vi "SVT Send Data to Waterfall for Octave.vi"(0 "waterfall ref":refnum<vi>, 1 "axis labels":T1, 5 "octave spectra":T6(array[cluster]) {"band power [dB EU]" format="%.2f"; "nominal frequencies [Hz]" format="%.2f"}, 7 "y0 and delta y":cluster{"y0":dbl, "delta y":dbl}={"y0"=0.0, "delta y"=1.0} {"delta y" format="%.2f"; "y0" format="%.2f"}, 9 "octave info":T2={"standard"=enum."ANSI S1.11", "bandwidth"=enum."1 octave", "low band"=0, "high band"=0, "weighting filter"=0, "dB reference"=0.0, "dB On"=FALSE, "unit label"="", "channel name"="", "description"="", "engineering units"=1, "custom label"="", "spectrum type"=enum."magnitude", "spectral density"=FALSE, "filters settled"=FALSE} {"engineering units" items=["custom..."=0, "V"=1, "A"=21, "C"=30, "pC"=31, "s"=32, "-"=29, "Pa"=2, "N"=20, "g"=3, "m/s^2"=4, "m/s"=5, "m"=6, "mm/s"=12, "mm"=13, "micron/s"=14, "micron"=15, "in/s^2"=7, "in/s"=8, "in"=9, "mil/s"=10, "mil"=11, "rad/s^2"=16, "rad/s"=17, "rad"=18, "deg/s^2"=26, "deg/s"=27, "deg"=28, "RPM"=22, "cycle/s^2"=23, "Hz"=24, "cycle"=25, "strain"=19]; "dB reference" format="%.2e"; "weighting filter" items=["Linear", "A-weighting", "B-weighting", "C-weighting", "ITU-R 468-4", "Dolby", "CCITT", "C-message", "Wb", "Wc", "Wd", "We", "Wf", "Wh", "Wj", "Wk", "Wm", "AES17 20 kHz lowpass", "AES17 40 kHz lowpass", "AES17 20 kHz highpass", "AES17 40 kHz highpass"]}, 11 "error in (no error)":errorcluster, 12 "settings":T7={"clear graph before redrawing (F)"=FALSE, "set baseline (F)"=FALSE, "baseline"=0.0, "autoscale (T)"=TRUE} {"baseline" format="%.2f"}, 13 "frontmost (T)":bool=TRUE) -> (4 "dup waterfall ref":refnum<vi>, 15 "error out":errorcluster)   [LabVIEW 2017]
doc: "Sends the waterfall data, or octave spectra, to the waterfall display."
uses:
  <vilib>/addons/Sound and Vibration/svt_Octave/subVIs/sv_Octave Info.ctl
  <vilib>/addons/_NISVFA/_Shared subVIs/Controls/svc_Octave Standard.ctl
  <vilib>/addons/_NISVFA/_Shared subVIs/Controls/svc_Weighting Filter Text Ring.ctl
  <vilib>/addons/_NISVFA/_Shared subVIs/Controls/svc_Engineering Units Text Ring.ctl
  <vilib>/addons/Sound and Vibration/compatibility/Waterfall/subVIs/sv_Waterfall for Octave Global.vi
  <vilib>/addons/Sound and Vibration/svt_Octave/SoundVib_Octave.lvlib
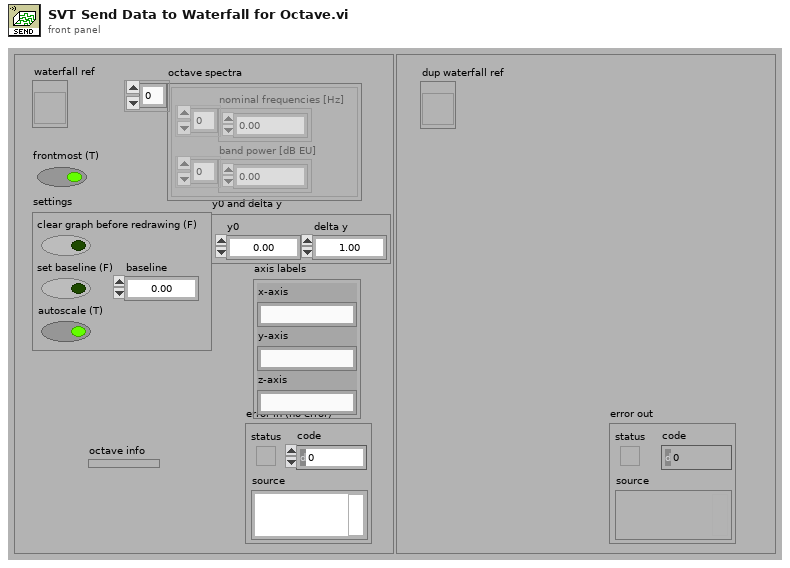
[diagram p1: front panel]
types:
  T1 = cluster{"x-axis":string, "y-axis":string, "z-axis":string}
  T2 = typedef "SoundVib_Octave.lvlib/sv_Octave Info.ctl" = cluster{"standard":T3, "bandwidth":enum16{"1 octave", "1/3 octave", "1/6 octave", "1/12 octave", "1/24 octave"}, "low band":i32, "high band":i32, "weighting filter":T4, "dB reference":dbl, "dB On":bool, "unit label":string, "channel name":string, "description":string, "engineering units":T5, "custom label":string, "spectrum type":enum16{"power", "magnitude"}, "spectral density":bool, "filters settled":bool}
  T3 = typedef "svc_Octave Standard.ctl" = enum16{"ANSI S1.11", "IEC 61260"}
  T4 = typedef "svc_Weighting Filter Text Ring.ctl" = u16
  T5 = typedef "svc_Engineering Units Text Ring.ctl" = u16
  T6 = cluster{"nominal frequencies [Hz]":dbl[], "band power [dB EU]":dbl[]}[]
  T7 = cluster{"clear graph before redrawing (F)":bool, "set baseline (F)":bool, "baseline":dbl, "autoscale (T)":bool}
  T8 = cluster{"f low":dbl, "f high":dbl, "midband":dbl}[]
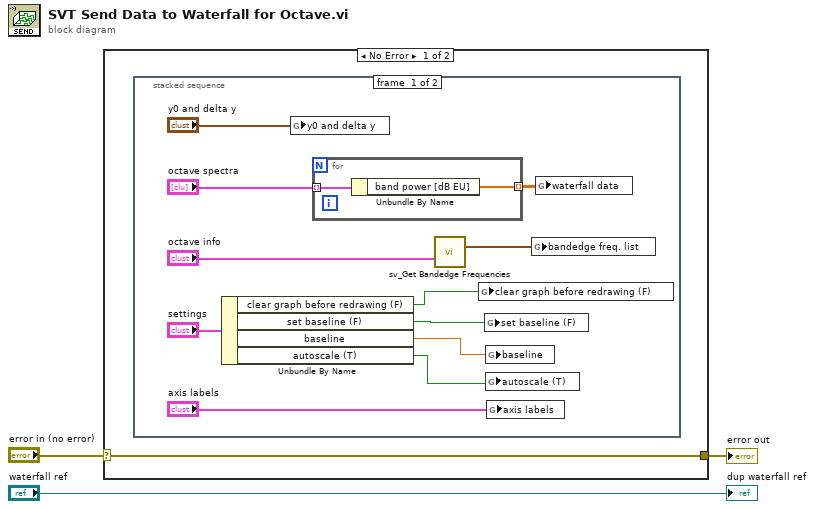
[diagram p0: block diagram]
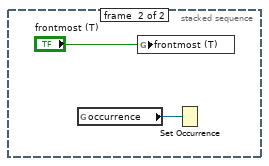
[diagram p2: hidden frame]
diagram:
  n1 = case shown="No Error" "error in (no error)" {
    selector: "error in (no error)" -> [w4 w20]
    tunnel: [w4 w20] -> w1
    frame No Error {
      n2 = stacked-sequence {
        frame #0 {
          n3 = Unbundle By Name("settings") -> ("clear graph before redrawing (F)"=w13:bool, "set baseline (F)"=w12:bool, "baseline"=w11:dbl, "autoscale (T)"=w10:bool)
          n4 = global write "sv_Waterfall for Octave Global.vi" "y0 and delta y"("y0 and delta y") -> ()
          n5 = for {
            tunnel: "octave spectra" -> [w17] mode=indexing
            tunnel: [w16] -> w8 mode=indexing
            n6 = Unbundle By Name(w17) -> ("band power [dB EU]"=w16:dbl[])
          }
          n7 = call <vilib>:"sv_Get Bandedge Frequencies.vi"("octave info"="octave info") -> ("bandedge frequencies [Hz]"=w7:T8)  [unwired: 13 in, 1 out]
          n8 = global write "sv_Waterfall for Octave Global.vi" "clear graph before redrawing (F)"(w13) -> ()
          n9 = global write "sv_Waterfall for Octave Global.vi" "set baseline (F)"(w12) -> ()
          n10 = global write "sv_Waterfall for Octave Global.vi" "baseline"(w11) -> ()
          n11 = global write "sv_Waterfall for Octave Global.vi" "autoscale (T)"(w10) -> ()
          n12 = global write "sv_Waterfall for Octave Global.vi" "axis labels"("axis labels") -> ()
          n13 = global write "sv_Waterfall for Octave Global.vi" "bandedge freq. list"(w7) -> ()
          n14 = global write "sv_Waterfall for Octave Global.vi" "waterfall data"(w8) -> ()
        }
        frame #1 {
          n15 = global read "sv_Waterfall for Octave Global.vi" "occurrence"() -> (w19:refnum<k4>)
          n16 = global write "sv_Waterfall for Octave Global.vi" "frontmost (T)"("frontmost (T)") -> ()
          n17 = Set Occurrence(w19) -> ()
        }
      }
    }
    frame Error {
    }
  }
  "error out" <- w1
  "dup waterfall ref" <- "waterfall ref"
